vi "sfkgas;lbv.vi"() -> ()   [LabVIEW 2020]
uses:
  <vilib>/numeric/Random Number (Range) U64.vi
  <vilib>/numeric/sub_Random U32.vi
panel:
  in  "stop":bool
  out "Array 4":i32[](array[numeric])
  out "Numeric":i32
  out "Reversed array":u64[](array[numeric])
  out "Array":u64[](array[numeric])
  in  "Fahrenheit":dbl
  out "Celsius":dbl
  out "LED":bool
  in  "Switch":bool
  out "Array 2":dbl[](array[numeric])
  in  "Array":dbl[](array[numeric])
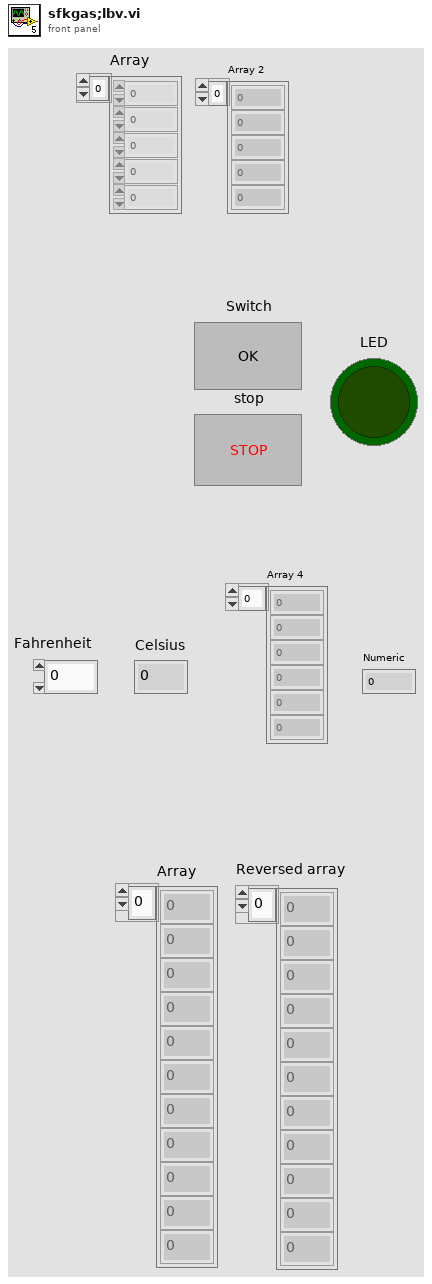
[diagram p1: front panel]
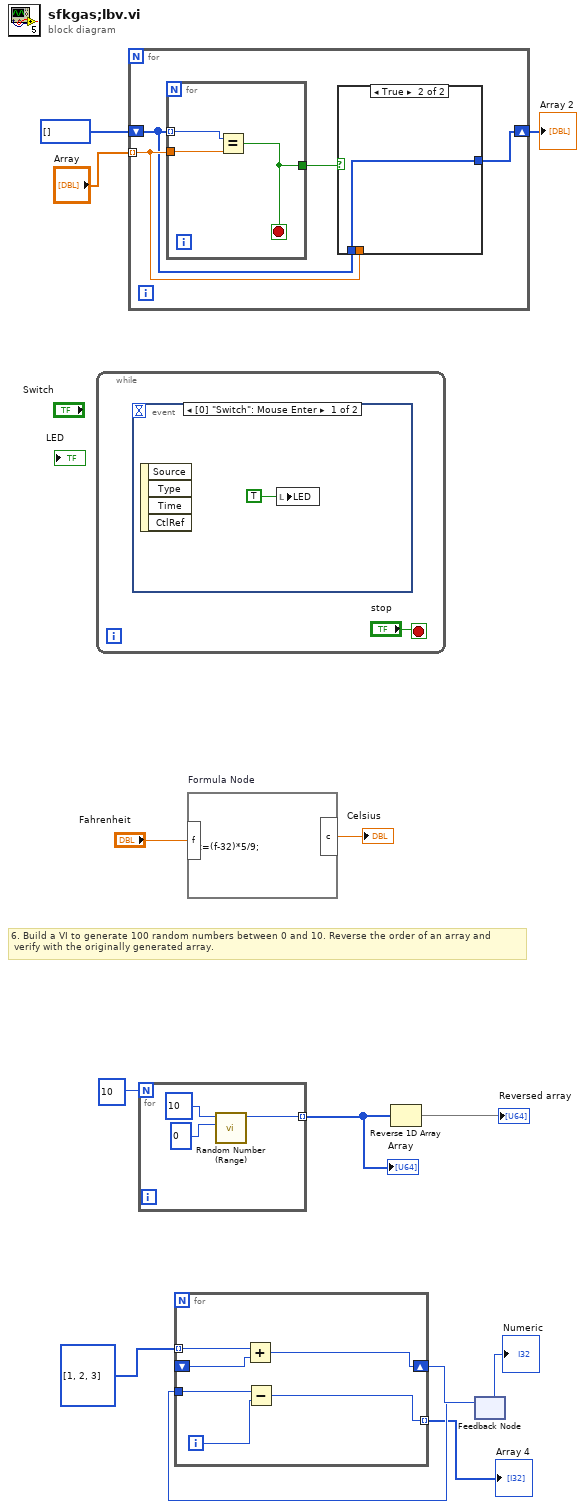
[diagram p0: block diagram]
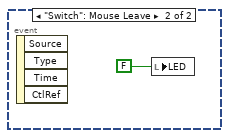
[diagram p2: hidden frame]
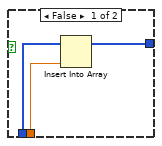
[diagram p3: hidden frame]
diagram:
  # "6.\tBuild a VI to generate 100 random numbers between 0 and 10. Reverse the order of an array and\n verify with the originally generated array."
  n1 = while {
    stop <- "stop" stop-if-true
    n2 = event shown="[0] \"Switch\": Mouse Enter" {
      selector: _ -> [_ _]
      dyn-events: _ -> [_ _]
      timeout: _ -> [_ _]
      event "Switch": Mouse Enter {
        n3 = event-data() -> ()  [unwired: 1 in, 4 out]
        n4 = local write "LED"(TRUE ("Boolean")) -> ()
      }
      event "Switch": Mouse Leave {
        n5 = event-data() -> ()  [unwired: 1 in, 4 out]
        n6 = local write "LED"(FALSE ("Boolean")) -> ()
      }
    }
  }
  n7 = for {
    tunnel: "Array" -> [w19] mode=indexing
    shift-right: [w16] -> w10
    shift-left: i32[] [] -> [w18]
    n8 = for {
      tunnel: w18 -> [w26] mode=indexing
      tunnel: w19 -> [w25]
      tunnel: [w24] -> w17
      stop <- w24 stop-if-true
      n9 = Equal?(x=w26, y=w25) -> (x = y?=w24:bool)
    }
    n10 = case shown="True" w17 {
      tunnel: w19 -> [w20 _]
      tunnel: w18 -> [w22 w23]
      tunnel: [w21 w23] -> w16
      frame False {
        n11 = Insert Into Array(array=w22, new element=w20) -> (w21:i32[])  [unwired: 1 in]
      }
      frame True {
      }
    }
  }
  "Array 2" <- w10
  n12 = for {
    N: 10 -> [_]
    tunnel: [w27] -> w5 mode=indexing
    n13 = call-poly <vilib>:"Random Number (Range).vi"("lower bound (0)"=u64 0, "upper bound (100)"=u64 10) -> ("number"=w27:u64)  [unwired: 9 in]
  }
  "Array" <- w5
  n14 = formula code="c=(f-32)*5/9;"("f"="Fahrenheit") -> ("c"=→"Celsius":dbl)
  n15 = Reverse 1D Array(array=w5) -> (reversed array=→"Reversed array":u64[])
  n16 = feedback #1() -> (w2:i32)  [unwired: 1 in]
  "Numeric" <- w2
  n17 = for {
    tunnel: i32[] [1, 2, 3] -> [w35] mode=indexing
    shift-right: [w33] -> w3
    shift-left: _ -> [w34]
    tunnel: w2 -> [w32]
    tunnel: [w30] -> w1 mode=indexing
    i -> [w31]
    n18 = Add(x=w35, y=w34) -> (x+y=w33:i32)
    n19 = Subtract(x=w32, y=w31) -> (x-y=w30:i32)
  }
  "Array 4" <- w1
  n20 = feedback-in #1(w3) -> ()
